vi "Base File Path.vi"() -> (3 "Paths Out":T1)   [LabVIEW 2016]
uses:
  File Paths.ctl
panel:
  in  "Paths":T1
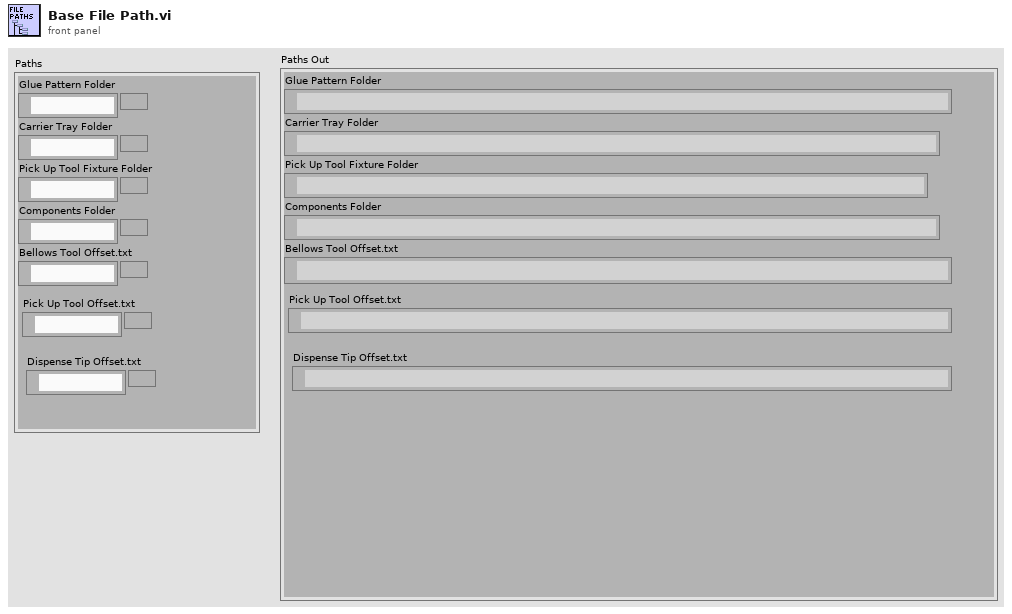
[diagram p1: front panel]
types:
  T1 = typedef "File Paths.ctl" = cluster{"Glue Pattern Folder":path, "Carrier Tray Folder":path, "Pick Up Tool Fixture Folder":path, "Components Folder":path, "Bellows Tool Offset.txt":path, "Pick Up Tool Offset.txt":path, "Dispense Tip Offset.txt":path}
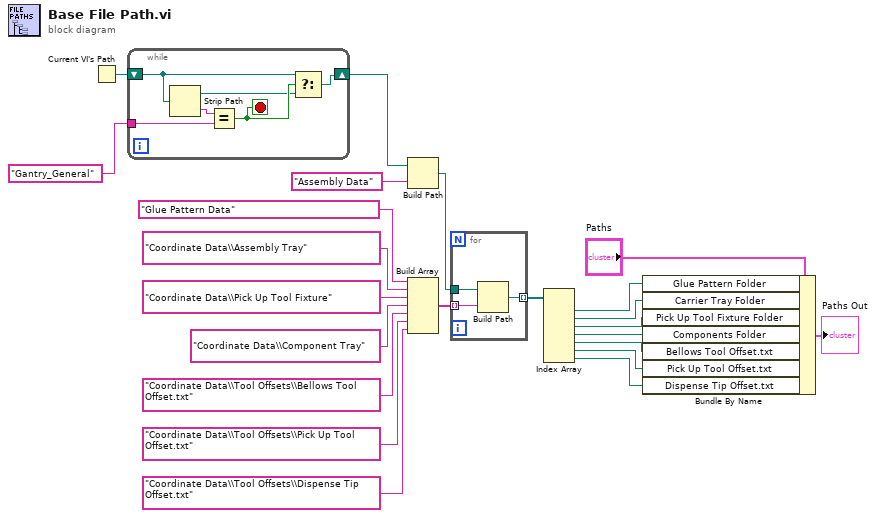
[diagram p0: block diagram]
diagram:
  n1 = Current VI's Path() -> (path=w23:path)
  n2 = while {
    shift-right: [w25] -> w19
    shift-left: w23 -> [w27]
    tunnel: "Gantry_General" -> [w24]
    stop <- w28 stop-if-true
    n3 = Strip Path(path=w27) -> (stripped path=w26:path, name=w29:string)
    n4 = Equal?(x=w29, y=w24) -> (x = y?=w28:bool)
    n5 = Select(t=w27, s=w28, f=w26) -> (s? t:f=w25:path)
  }
  n6 = Build Path(base path=w19, name or relative path="Assembly Data") -> (appended path=w17:path)
  n7 = Build Array("Glue Pattern Data", "Coordinate Data\\Assembly Tray", "Coordinate Data\\Pick Up Tool Fixture", "Coordinate Data\\Component Tray" ("element"), "Coordinate Data\\Tool Offsets\\Bellows Tool Offset.txt", "Coordinate Data\\Tool Offsets\\Pick Up Tool Offset.txt", "Coordinate Data\\Tool Offsets\\Dispense Tip Offset.txt") -> (w9:string[])
  n8 = for {
    tunnel: w17 -> [w32]
    tunnel: [w31] -> w21 mode=indexing
    tunnel: w9 -> [w30] mode=indexing
    n9 = Build Path(base path=w32, name or relative path=w30) -> (appended path=w31:path)
  }
  n10 = Index Array(array=w21) -> (element #1=w8:path, element #2=w7:path, element #3=w6:path, element #4=w5:path, element #5=w4:path, element #6=w3:path, element #7=w2:path)  [unwired: 7 in]
  n11 = Bundle By Name(cluster="Paths", "Glue Pattern Folder"=w8, "Carrier Tray Folder"=w7, "Pick Up Tool Fixture Folder"=w6, "Components Folder"=w5, "Bellows Tool Offset.txt"=w4, "Pick Up Tool Offset.txt"=w3, "Dispense Tip Offset.txt"=w2) -> (→"Paths Out":T1)
